vi "User Event-Title Bar-Mouse Down.vi"(8 "Error In":errorcluster, 11 "Appearance Actor in":refnum<class "Appearance Actor.lvclass">) -> (0 "Error Out":errorcluster, 3 "Appearance Actor out":refnum<class "Appearance Actor.lvclass">)   [LabVIEW 2021, in "Appearance Actor.lvlib" / "Appearance Actor.lvclass"]
doc: "Handles Mouse Down Event on Title Bar. By Default, call win32 API to move the window. Override this method to change its behavior."
uses:
  Appearance Actor.lvclass
  Appearance Actor.lvclass/Appearance Actor.ctl
  Windows/System32/user32.dll
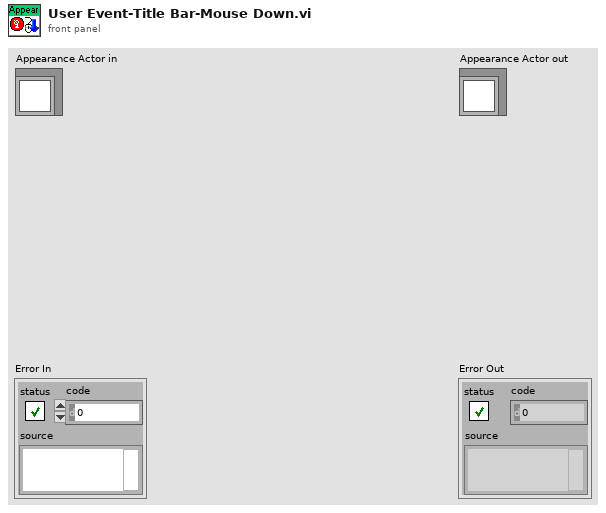
[diagram p1: front panel]
types:
  T1 = typedef "Appearance Actor.lvlib/Appearance Actor.lvclass/Docking State--enum.ctl" = enum16{"Not A SubPanel", "Docked", "UnDocked"}
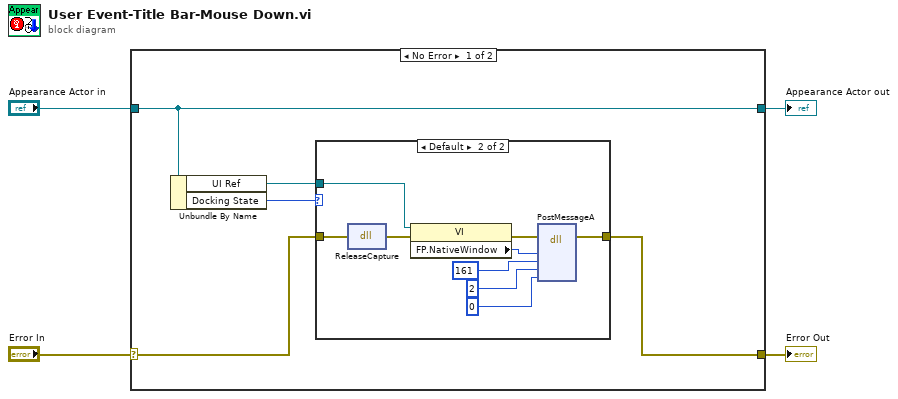
[diagram p0: block diagram]
diagram:
  n1 = case shown="No Error" "Error In" {
    selector: "Error In" -> [w9 w21]
    tunnel: [w8 w21] -> w3
    tunnel: [w7 w20] -> w1
    tunnel: "Appearance Actor in" -> [w7 w20]
    frame No Error {
      n2 = Unbundle By Name(w7) -> ("UI Ref"=w6:refnum<vi>, "Docking State"=w5:T1)
      n3 = case shown="Default" w5 {
        tunnel: w9 -> [w10 w14]
        tunnel: [w10 w13] -> w8
        tunnel: w6 -> [_ w11]
        frame "Docked" {
        }
        frame Default {
          n4 = dll-call lib="C:/Windows/System32/user32.dll" fn="ReleaseCapture"(error in=w14) -> (error out=w19:errorcluster)  [unwired: 3 in, 1 out]
          n5 = property class="VI"(reference=w11, error in=w19) -> (error out=w12:errorcluster, "FP.NativeWindow"=w18:u64)  [unwired: 1 out]
          n6 = dll-call lib="C:/Windows/System32/user32.dll" fn="PostMessageA"(error in=w12, "arg1"=w18, "arg2"=161, "arg3"=2, "arg4"=0) -> (error out=w13:errorcluster)  [unwired: 7 in, 1 out]
        }
      }
    }
    frame Error {
    }
  }
  "Error Out" <- w3
  "Appearance Actor out" <- w1
